vi "5492_AutoSpitNoPID.vi"   [LabVIEW 2017]
uses:
  5492_SpitButton.vi
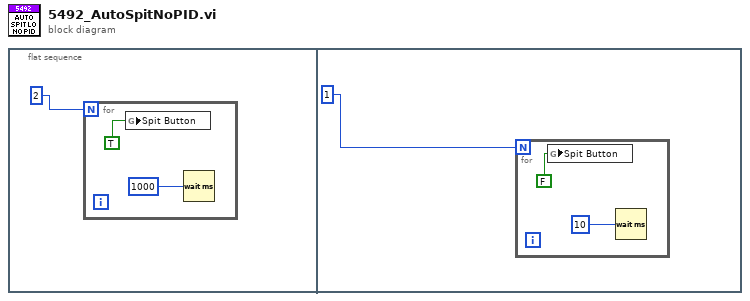
[diagram p0: block diagram]
diagram:
  n1 = flat-sequence {
    frame #0 {
      n2 = for {
        N: 2 -> [_]
        n3 = global write "5492_SpitButton.vi" "Spit Button"(TRUE ("Lo")) -> ()
        n4 = Wait (ms)(milliseconds to wait=u32 1000) -> ()  [unwired: 1 out]
      }
    }
    frame #1 {
      n5 = for {
        N: 1 -> [_]
        n6 = global write "5492_SpitButton.vi" "Spit Button"(FALSE ("Lo")) -> ()
        n7 = Wait (ms)(milliseconds to wait=u32 10) -> ()  [unwired: 1 out]
      }
    }
  }
